vi "Notification by Reference.vi"(0 "Notifier In":refnum<notifier>, 2 "Temperature & Reset":bool, 7 "Image In":T1, 11 "Error In":errorcluster, 12 "Reset":refnum<vi>, 13 "Temperature In Range":refnum<vi>, 14 "High Temperature":refnum<vi>) -> (4 "Notifier out":refnum<notifier>, 15 "Error out":errorcluster)   [LabVIEW 2016]
uses:
  <vilib>/vision/Image Controls.llb/IMAQ Image.ctl
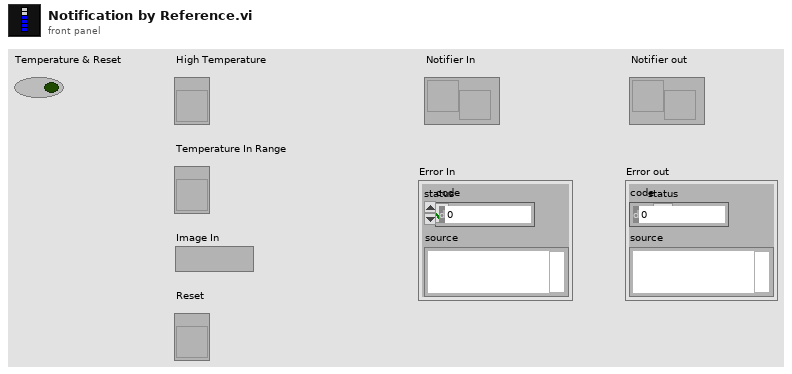
[diagram p1: front panel]
types:
  T1 = typedef "IMAQ Image.ctl" = refnum<image>
  T2 = enum8{"Enabled", "Disabled", "Disabled and Grayed Out"}
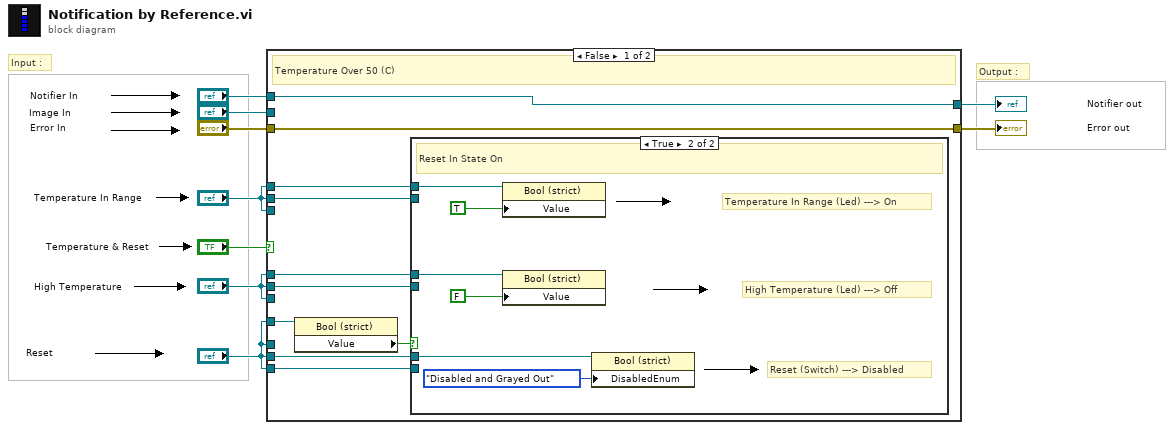
[diagram p0: block diagram]
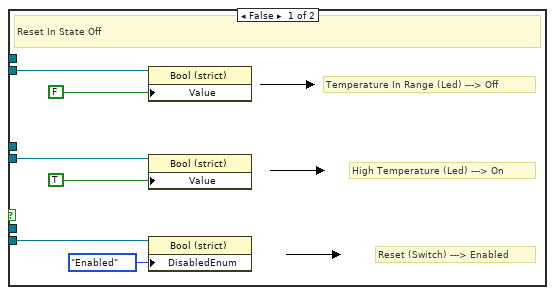
[diagram p2: hidden frame]
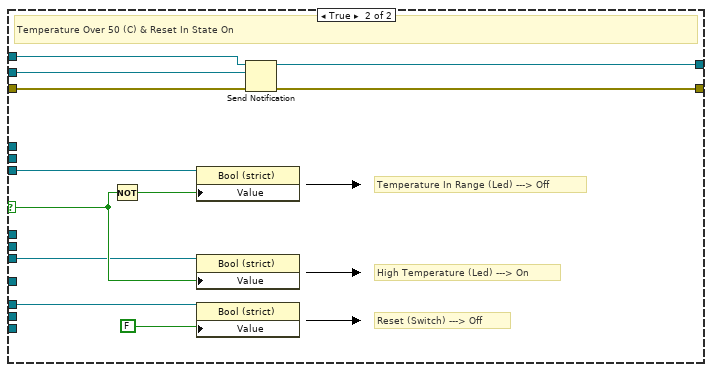
[diagram p3: hidden frame]
diagram:
  # "Input :"
  # "Output :"
  n1 = case shown="False" "Temperature & Reset" {
    selector: "Temperature & Reset" -> [_ w36]
    tunnel: "Notifier In" -> [w18 w42]
    tunnel: [w19 w41] -> w5
    tunnel: "Error In" -> [w19 w40]
    tunnel: [w18 w39] -> w7
    tunnel: "Image In" -> [_ w38]
    tunnel: "High Temperature" -> [w16 _]
    tunnel: "Temperature In Range" -> [w15 _]
    tunnel: "Reset" -> [w14 _]
    tunnel: "High Temperature" -> [w13 _]
    tunnel: "Temperature In Range" -> [w12 _]
    tunnel: "Reset" -> [w11 _]
    tunnel: "Reset" -> [w10 _]
    tunnel: "Reset" -> [_ w34]
    tunnel: "High Temperature" -> [_ w33]
    tunnel: "Temperature In Range" -> [_ w32]
    frame False {
      # "Temperature Over 50 (C)"
      n2 = property class="Bool (strict)"(reference=w10) -> ("Value"=w17:bool)  [unwired: 1 in, 2 out]
      n3 = case shown="True" w17 {
        tunnel: w16 -> [w22 _]
        tunnel: w15 -> [w21 _]
        tunnel: w14 -> [w20 _]
        tunnel: w13 -> [_ w28]
        tunnel: w12 -> [_ w27]
        tunnel: w11 -> [_ w26]
        frame False {
          # "Reset (Switch) ---> Enabled"
          # "High Temperature (Led) ---> On"
          # "Temperature In Range (Led) ---> Off"
          # "Reset In State Off"
          n4 = property class="Bool (strict)"(reference=w21, "Value"=FALSE ("Temperature In Range")) -> ()  [unwired: 1 in, 2 out]
          n5 = property class="Bool (strict)"(reference=w22, "Value"=TRUE ("High Temperature")) -> ()  [unwired: 1 in, 2 out]
          n6 = property on="Property Node" class="Bool (strict)"(reference=w20, "DisabledEnum"=T2."Enabled" ("Disabled")) -> ()  [unwired: 1 in, 2 out]
        }
        frame True {
          # "Reset (Switch) ---> Disabled"
          # "High Temperature (Led) ---> Off"
          # "Temperature In Range (Led) ---> On"
          # "Reset In State On"
          n7 = property class="Bool (strict)"(reference=w27, "Value"=TRUE ("Temperature In Range")) -> ()  [unwired: 1 in, 2 out]
          n8 = property class="Bool (strict)"(reference=w28, "Value"=FALSE ("High Temperature")) -> ()  [unwired: 1 in, 2 out]
          n9 = property on="Property Node" class="Bool (strict)"(reference=w26, "DisabledEnum"=T2."Disabled and Grayed Out" ("Disabled")) -> ()  [unwired: 1 in, 2 out]
        }
      }
    }
    frame True {
      # "Reset (Switch) ---> Off"
      # "High Temperature (Led) ---> On"
      # "Temperature In Range (Led) ---> Off"
      # "Temperature Over 50 (C) & Reset In State On"
      n10 = Not(x=w36) -> (.not. x?=w35:bool)
      n11 = property class="Bool (strict)"(reference=w32, "Value"=w35) -> ()  [unwired: 1 in, 2 out]
      n12 = property class="Bool (strict)"(reference=w33, "Value"=w36) -> ()  [unwired: 1 in, 2 out]
      n13 = property class="Bool (strict)"(reference=w34, "Value"=FALSE ("Reset")) -> ()  [unwired: 1 in, 2 out]
      n14 = Send Notification(notification=w38, notifier=w42, error in (no error)=w40) -> (notifier out=w39:refnum<notifier>, error out=w41:errorcluster)
    }
  }
  "Notifier out" <- w7
  "Error out" <- w5
